vi "Wait For Previous.vi"(8 "error in (no error)":errorcluster, 9 "timeout in ms (0)":i32 format="%d ms", 11 "Transfer Group in":refnum<class "Transfer Group.lvclass">) -> (0 "error out":errorcluster, 2 "ready":bool, 3 "Transfer Group out":refnum<class "Transfer Group.lvclass">)   [LabVIEW 2017, in "DSF Core.lvlib" / "Transfer Group.lvclass"]
uses:
  Transfer Group.lvclass
  Transfer Group.lvclass/Transfer Group.ctl
  Timing/Timing.lvclass/Timing.ctl
  Read Return FIFO.vi
  Errors.vi
  Return Timeout Error.vi
  Increment Late Count.vi
  Invalid Iteration Error.vi
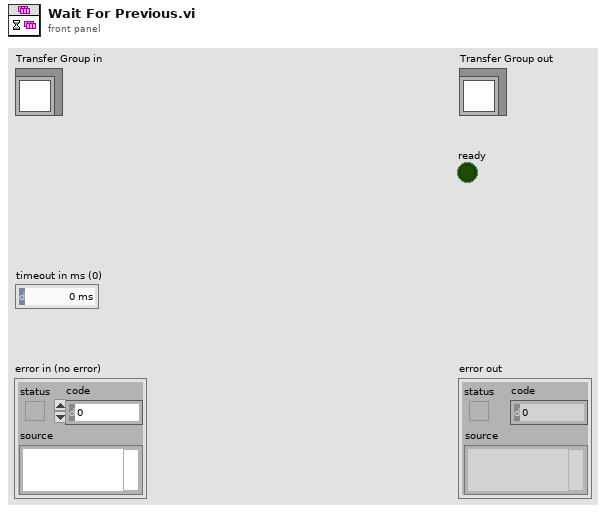
[diagram p1: front panel]
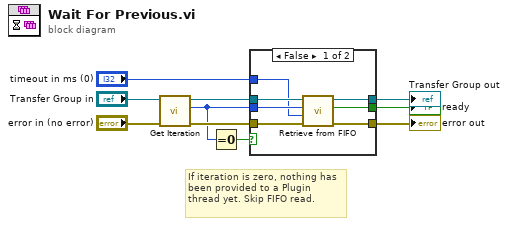
[diagram p0: block diagram]
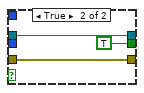
[diagram p2: hidden frame]
diagram:
  # "If iteration is zero, nothing has been provided to a Plugin thread yet. Skip FIFO read."
  n1 = call "Get Iteration.vi"("error in (no error)"="error in (no error)", "Transfer Group in"="Transfer Group in") -> ("error out"=w9:errorcluster, "iteration"=w8:u64, "Transfer Group out"=w7:refnum<class "Transfer Group.lvclass">)  [unwired: 7 in]
  n2 = Equal To 0?(x=w8) -> (x = 0?=w10:bool)
  n3 = case shown="False" w10 {
    tunnel: w9 -> [w17 w20]
    tunnel: [w16 w18] -> w3
    tunnel: [w15 w20] -> w4
    tunnel: w7 -> [w14 w18]
    tunnel: w8 -> [w13 _]
    tunnel: [w11 TRUE ("iteration valid?")] -> w2
    tunnel: "timeout in ms (0)" -> [w12 _]
    frame False {
      n4 = call "Retrieve from FIFO.vi"("error in (no error)"=w17, "timeout in ms (0)"=w12, "expected iteration"=w13, "Transfer Group in"=w14) -> ("error out"=w15:errorcluster, "ready"=w11:bool, "Transfer Group out"=w16:refnum<class "Transfer Group.lvclass">)  [unwired: 5 in]
    }
    frame True {
    }
  }
  "error out" <- w4
  "Transfer Group out" <- w3
  "ready" <- w2
